vi "Ramp up.vi"(10 "time":dbl) -> (2 "Power Out":dbl)   [LabVIEW 2017]
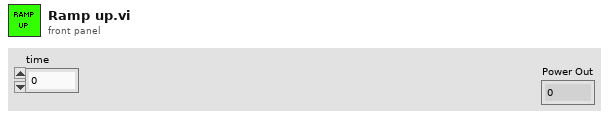
[diagram p1: front panel]
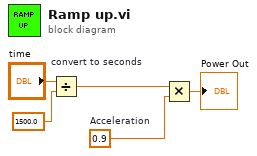
[diagram p0: block diagram]
diagram:
  w5 = 0.9  # Acceleration
  n1 = Divide "convert to seconds"(x="time", y=1500.0 ("time")) -> (x/y=w4:dbl)
  n2 = Multiply(x=w4, y=w5) -> (x*y=→"Power Out":dbl)
